vi "LS370_read_only_Splitt_cluster.vi"(0 "Lakeshore 370 read only":T3) -> (1 "Lakeshore 370 read only Status":T2, 2 "Lakeshore 370 read only Control":T1)   [LabVIEW 2019]
uses:
  LS370/Monitor/LS370_only_readout_cluster.ctl
  LS370/LS370_read_only_status.ctl
  LS370/LS370_read_only_control.ctl
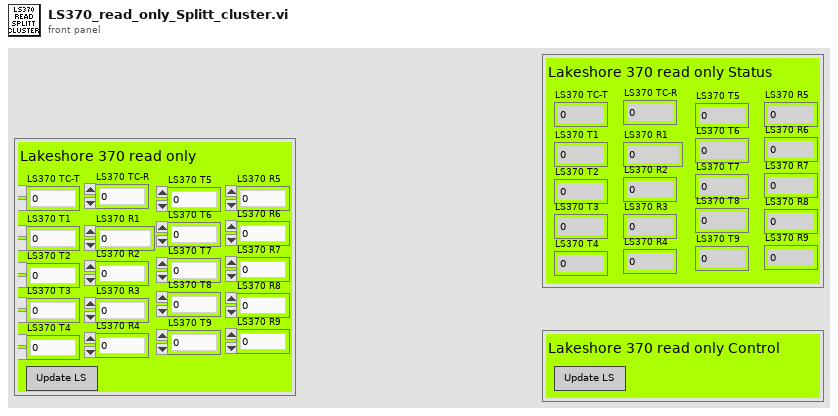
[diagram p1: front panel]
types:
  T1 = typedef "LS370_read_only_control.ctl" = cluster{"Update Lakeshores":bool}
  T2 = typedef "LS370_read_only_status.ctl" = cluster{"LS370 T1":dbl, "LS370 T2":dbl, "LS370 T3":dbl, "LS370 T4":dbl, "LS370 T5":dbl, "LS370 R1":dbl, "LS370 R2":dbl, "LS370 R3":dbl, "LS370 R4":dbl, "LS370 R5":dbl, "LS370 T6":dbl, "LS370 T7":dbl, "LS370 T8":dbl, "LS370 T9":dbl, "LS370 R6":dbl, "LS370 R7":dbl, "LS370 R8":dbl, "LS370 R9":dbl, "LS370 TC-T":dbl, "LS370 TC-R":dbl}
  T3 = typedef "LS370_only_readout_cluster.ctl" = cluster{"LS370 T1":dbl, "LS370 T2":dbl, "LS370 T3":dbl, "LS370 T4":dbl, "LS370 T5":dbl, "LS370 R1":dbl, "LS370 R2":dbl, "LS370 R3":dbl, "LS370 R4":dbl, "LS370 R5":dbl, "LS370 T6":dbl, "LS370 T7":dbl, "LS370 T8":dbl, "LS370 T9":dbl, "LS370 R6":dbl, "LS370 R7":dbl, "LS370 R8":dbl, "LS370 R9":dbl, "LS370 TC-T":dbl, "LS370 TC-R":dbl, "Update Lakeshores":bool}
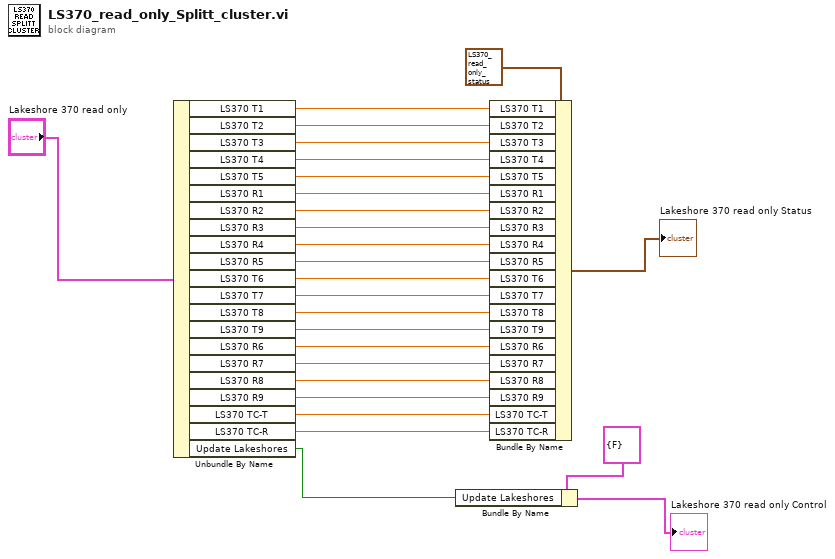
[diagram p0: block diagram]
diagram:
  n1 = Unbundle By Name("Lakeshore 370 read only") -> ("LS370 T1"=w23:dbl, "LS370 T2"=w22:dbl, "LS370 T3"=w21:dbl, "LS370 T4"=w20:dbl, "LS370 T5"=w19:dbl, "LS370 R1"=w18:dbl, "LS370 R2"=w17:dbl, "LS370 R3"=w16:dbl, "LS370 R4"=w15:dbl, "LS370 R5"=w14:dbl, "LS370 T6"=w13:dbl, "LS370 T7"=w12:dbl, "LS370 T8"=w11:dbl, "LS370 T9"=w10:dbl, "LS370 R6"=w9:dbl, "LS370 R7"=w8:dbl, "LS370 R8"=w7:dbl, "LS370 R9"=w6:dbl, "LS370 TC-T"=w5:dbl, "LS370 TC-R"=w4:dbl, "Update Lakeshores"=w1:bool)
  n2 = Bundle By Name(cluster=T1 {"Update Lakeshores"=FALSE} ("Lakeshore 370 read only Control"), "Update Lakeshores"=w1) -> (→"Lakeshore 370 read only Control":T1)
  n3 = Bundle By Name(cluster=T2 {"LS370 T1"=0.0, "LS370 T2"=0.0, "LS370 T3"=0.0, "LS370 T4"=0.0, "LS370 T5"=0.0, "LS370 R1"=0.0, "LS370 R2"=0.0, "LS370 R3"=0.0, "LS370 R4"=0.0, "LS370 R5"=0.0, "LS370 T6"=0.0, "LS370 T7"=0.0, "LS370 T8"=0.0, "LS370 T9"=0.0, "LS370 R6"=0.0, "LS370 R7"=0.0, "LS370 R8"=0.0, "LS370 R9"=0.0, "LS370 TC-T"=0.0, "LS370 TC-R"=0.0} ("Lakeshore 370 read only Status 2"), "LS370 T1"=w23, "LS370 T2"=w22, "LS370 T3"=w21, "LS370 T4"=w20, "LS370 T5"=w19, "LS370 R1"=w18, "LS370 R2"=w17, "LS370 R3"=w16, "LS370 R4"=w15, "LS370 R5"=w14, "LS370 T6"=w13, "LS370 T7"=w12, "LS370 T8"=w11, "LS370 T9"=w10, "LS370 R6"=w9, "LS370 R7"=w8, "LS370 R8"=w7, "LS370 R9"=w6, "LS370 TC-T"=w5, "LS370 TC-R"=w4) -> (→"Lakeshore 370 read only Status":T2)
